vi "Load Step Classes.vi"(8 "error in (no error)":errorcluster, 11 "Step Classes Folder Path":path) -> (0 "error out":errorcluster, 3 "Step Class Library":T1)   [LabVIEW 2015, in "Configuration Tool.lvlib"]
uses:
  Configuration Tool.lvlib
  Controls/StepClassLibrary.ctl
  Prototype/classes/Step/Config/Step Config.lvclass
  <vilib>/Utility/error.llb/Error Cluster From Error Code.vi
  <vilib>/ErrorRing/Error Ring.xnode
  <vilib>/NI/Configuration Framework/class discovery singleton/class discovery singleton.lvlib
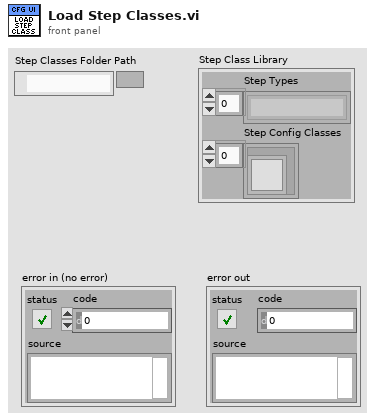
[diagram p1: front panel]
types:
  T1 = typedef "Configuration Tool.lvlib/StepClassLibrary.ctl" = cluster{"Step Types":string[], "Step Config Classes":refnum<class "Step Config.lvclass">[]}
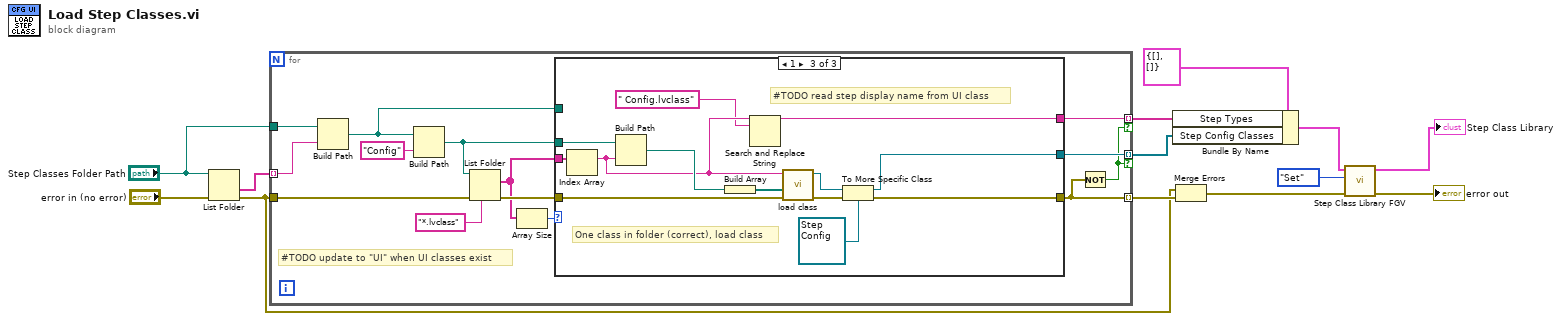
[diagram p0: block diagram]
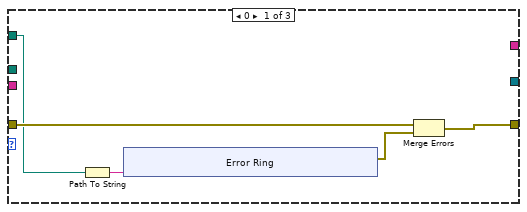
[diagram p2: hidden frame]
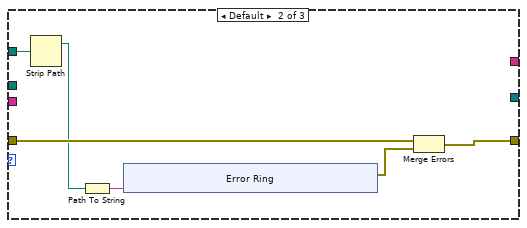
[diagram p3: hidden frame]
diagram:
  n1 = List Folder(path="Step Classes Folder Path", error in="error in (no error)") -> (folder names=w11:string[], error out=w9:errorcluster)  [unwired: 2 in, 2 out]
  n2 = for {
    tunnel: [w15] -> w6 mode=indexing if=w14
    tunnel: w11 -> [w25] mode=indexing
    tunnel: "Step Classes Folder Path" -> [w26]
    tunnel: w9 -> [w27]
    tunnel: [w20] -> w13 mode=indexing
    tunnel: [w16] -> w7 mode=indexing if=w14
    # "#TODO update to \"UI\" when UI classes exist"
    n3 = Build Path(base path=w26, name or relative path=w25) -> (appended path=w17:path)
    n4 = Build Path(base path=w17, name or relative path="Config") -> (appended path=w21:path)
    n5 = List Folder(path=w21, pattern="*.lvclass", error in=w27) -> (filenames=w19:string[], error out=w23:errorcluster)  [unwired: 1 in, 2 out]
    n6 = Array Size(array=w19) -> (size(s)=w18:i32)
    n7 = case shown="1" w18 {
      tunnel: w23 -> [w32 w45 w62]
      tunnel: w21 -> [_ _ w61]
      tunnel: w19 -> [_ _ w60]
      tunnel: [w31 w44 w55] -> w20
      tunnel: w17 -> [w30 w43 _]
      tunnel: [_ _ w54] -> w16
      tunnel: [_ _ w53] -> w15
      frame 0 {
        n8 = Path To String(path=w30) -> (string=w29:string)
        n9 = xnode "Error Ring"("parameter 0"=w29) -> ("error out"=w28:errorcluster)
        n10 = Merge Errors(w32, w28) -> (w31:errorcluster)
      }
      frame Default {
        n11 = Strip Path(path=w43) -> (stripped path=w42:path)  [unwired: 1 out]
        n12 = Path To String(path=w42) -> (string=w41:string)
        n13 = xnode "Error Ring"("parameter 0"=w41) -> ("error out"=w40:errorcluster)
        n14 = Merge Errors(w45, w40) -> (w44:errorcluster)
      }
      frame 1 {
        # "#TODO read step display name from UI class"
        # "One class in folder (correct), load class"
        n15 = Index Array(array=w60) -> (element=w57:string)  [unwired: 1 in]
        n16 = Build Path(base path=w61, name or relative path=w57) -> (appended path=w59:path)
        n17 = Build Array(w59) -> (w58:path[])
        n18 = Search and Replace String(input string=w57, search string=" Config.lvclass") -> (result string=w54:string)  [unwired: 6 in, 3 out]
        n19 = call <vilib>:"load class.vi"("error in"=w62, "available class paths"=w58, "Class Name"=w57) -> ("error out"=w63:errorcluster, "Object Out"=w65:refnum<class>)  [unwired: 7 in]
        n20 = To More Specific Class(target class=refnum<class "Step Config.lvclass"> refnum ("Step Config.lvclass"), reference=w65, error in=w63) -> (specific class reference=w53:refnum<class "Step Config.lvclass">, error out=w55:errorcluster)
      }
    }
    n21 = Not(x=w20) -> (.not. x?=w14:bool)
  }
  n22 = Bundle By Name(cluster=T1 {"Step Types"=[], "Step Config Classes"=[]}, "Step Types"=w7, "Step Config Classes"=w6) -> (w2:T1)
  n23 = Merge Errors(w9, w13) -> (w4:errorcluster)
  n24 = call "Step Class Library FGV.vi"("error in (no error)"=w4, "Action"=enum16{"Set", "Get"}."Set", "Step Type Class Library"=w2) -> ("error out"=→"error out":errorcluster, "Step Type Class Library out"=→"Step Class Library":T1)  [unwired: 7 in]
